vi "Add Layers to Top of Icon.vi"(10 "User layers":T1[](array[typedef]), 11 "Icon.lvclass in":refnum<class "Icon.lvclass">) -> (3 "Icon.lvclass out":refnum<class "Icon.lvclass">)   [LabVIEW 2020, in "Message Maker.lvlib"]
uses:
  Message Maker.lvlib
  <vilib>/LabVIEW Icon API/lv_icon/Controls/LayerType.ctl
  <vilib>/LabVIEW Icon API/lv_icon/Classes/Layer/Layer.lvclass
  <vilib>/LabVIEW Icon API/lv_icon/Controls/Layer.ctl
  <vilib>/LabVIEW Icon API/lv_icon/Classes/Icon/Icon.lvclass
  <vilib>/picture/picture.llb/imagedata.ctl
  <vilib>/Utility/miscctls.llb/LVPoint32TypeDef.ctl
  <vilib>/LabVIEW Icon API/API_User Layer Data.ctl
  <vilib>/LabVIEW Icon API/LabVIEW Icon API.lvlib
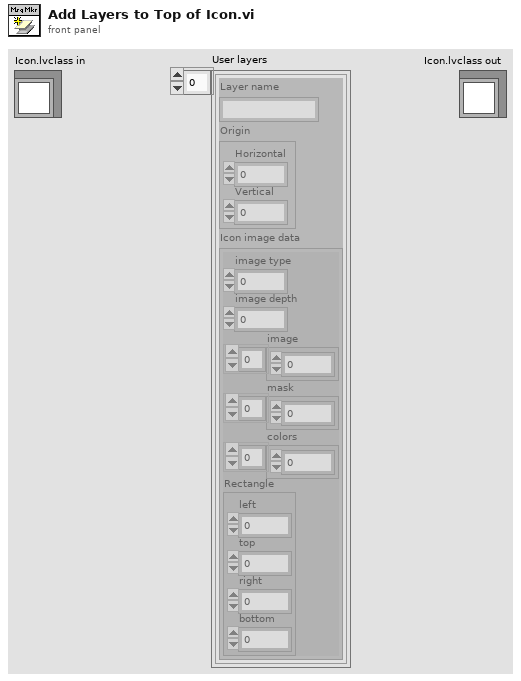
[diagram p1: front panel]
types:
  T1 = typedef "LabVIEW Icon API.lvlib/API_User Layer Data.ctl" = cluster{"Layer name":string, "Origin":T2, "Icon image data":T3}
  T2 = typedef "LVPoint32TypeDef.ctl" = cluster{"Horizontal":i32, "Vertical":i32}
  T3 = typedef "imagedata.ctl" = cluster{"image type":i32, "image depth":i32, "image":u8[], "mask":u8[], "colors":u32[], "Rectangle":cluster{"left":i16, "top":i16, "right":i16, "bottom":i16}}
  T4 = typedef "Layer.ctl" = cluster{"LayerIcon":picture, "LayerName":string, "Opacity":u8, "Visibility?":bool}
  T5 = typedef "LayerType.ctl" = enum16{"Graphic", "Text", "Tool", "Graphic Drop"}
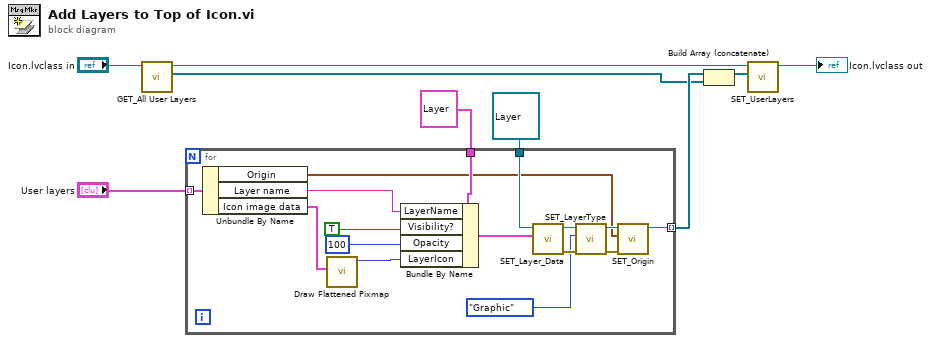
[diagram p0: block diagram]
diagram:
  n1 = call-dynamic "GET_All User Layers.vi"("Icon.lvclass in"="Icon.lvclass in") -> ("User Layer"=w3:refnum<class "Layer.lvclass">[], "Icon.lvclass out"=w1:refnum<class "Icon.lvclass">)  [unwired: 8 in, 1 out]
  n2 = for {
    tunnel: "User layers" -> [w25] mode=indexing
    tunnel: T4 {"LayerIcon"=bytes[0], "LayerName"="", "Opacity"=0, "Visibility?"=FALSE} ("Data") -> [w17]
    tunnel: refnum<class "Layer.lvclass"> refnum ("Layer.lvclass in") -> [w16]
    tunnel: [w12] -> w4 mode=indexing
    n3 = Unbundle By Name(w25) -> ("Origin"=w14:T2, "Layer name"=w18:string, "Icon image data"=w11:T3)
    n4 = call <vilib>:"Draw Flattened Pixmap.vi"("image data"=w11) -> ("new picture"=w10:picture)  [unwired: 8 in]
    n5 = Bundle By Name(cluster=w17, "LayerName"=w18, "Visibility?"=TRUE, "Opacity"=u8 100, "LayerIcon"=w10) -> (w21:T4)
    n6 = call-dynamic "SET_Layer_Data.vi"("Data"=w21, "Layer.lvclass in"=w16) -> ("error out"=w22:errorcluster, "Layer.lvclass out"=w20:refnum<class "Layer.lvclass">)  [unwired: 2 in, 6 out]
    n7 = call-dynamic "SET_LayerType.vi"("error in (no error)"=w22, "Type"=LayerType."Graphic", "Layer.lvclass in"=w20) -> ("error out"=w13:errorcluster, "Layer.lvclass out"=w15:refnum<class "Layer.lvclass">)  [unwired: 7 out]
    n8 = call-dynamic "SET_Origin.vi"("error in (no error)"=w13, "Point32"=w14, "Layer.lvclass in"=w15) -> ("Layer.lvclass out"=w12:refnum<class "Layer.lvclass">)  [unwired: 7 in, 1 out]
  }
  n9 = Build Array (concatenate)(w4, w3) -> (w2:refnum<class "Layer.lvclass">[])
  n10 = call-dynamic "SET_UserLayers.vi"("Layers"=w2, "Icon.lvclass in"=w1) -> ("Icon.lvclass out"=→"Icon.lvclass out":refnum<class "Icon.lvclass">)  [unwired: 8 in, 1 out]
